vi "Send Core.vi"(6 "Severity Code (info)":T1=enum."info", 8 "Error In":errorcluster, 9 "Message Content":string, 10 "Message Tag":string, 11 "CS++RTMessageLogger in":refnum<class "CS++RTMessageLogger.lvclass">) -> (0 "Error Out":errorcluster, 3 "CS++RTMessageLogger out":refnum<class "CS++RTMessageLogger.lvclass">)   [LabVIEW 2014, in "CS++RTClasses.lvlib" / "CS++RTMessageLogger.lvclass"]
doc: "Send mesage to message logger."
uses:
  CS++RTMessageLogger.lvclass
  CSPP_Core/Libraries/Base/Severity.ctl
  <vilib>/NI_Real-Time Target Support.lvlib
  CSPP_Core/Libraries/Base/CS++Base.lvlib
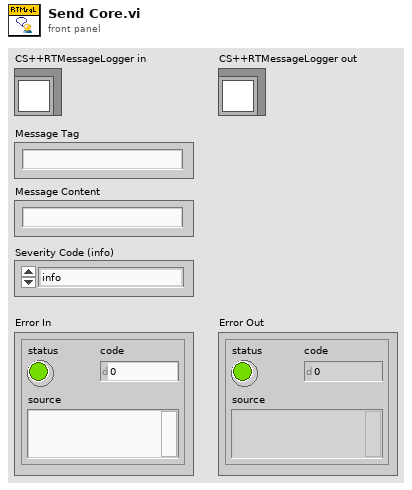
[diagram p1: front panel]
types:
  T1 = typedef "CS++Base.lvlib/Severity.ctl" = enum16{"emergency", "alert", "critical", "error", "warning", "notice", "info", "debug"}
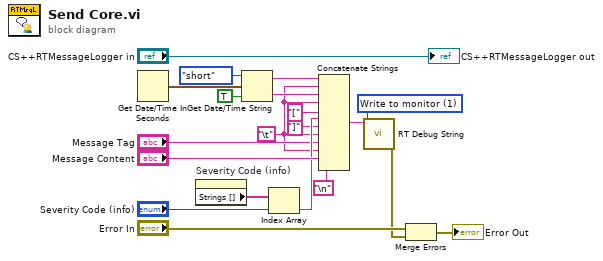
[diagram p0: block diagram]
diagram:
  w1 = "\t"
  w18 = u16 1 items=["Write to serial", "Write to monitor"] ("Interface")
  n1 = Get Date/Time In Seconds() -> (seconds since 1Jan1904=w9:timestamp)
  n2 = property on="Severity Code (info)" class="Enum (strict)"() -> ("Strings []"=w17:string[])  [unwired: 2 in, 2 out]
  n3 = Get Date/Time String(date format (0)=enum16{"short", "long", "abbreviated"}."short", seconds (now)=w9, want seconds? (F)=TRUE) -> (date string=w7:string, time string=w6:string)
  n4 = Index Array(array=w17, index="Severity Code (info)") -> (element=w5:string)
  n5 = Concatenate Strings(w7, w1, w6, w1, "[" ("string"), w5, "]" ("string"), w1, "Message Tag", w1, "Message Content", "\n") -> (w15:string)
  n6 = call <vilib>:"RT Debug String.vi"("Interface"=w18, "String to write"=w15) -> ("error out"=w12:errorcluster)  [unwired: 9 in]
  n7 = Merge Errors("Error In", w12) -> (→"Error Out":errorcluster)
  "CS++RTMessageLogger out" <- "CS++RTMessageLogger in"
